vi "rs3 release frame.vi"(8 "error in (no error)":errorcluster, 11 "Frame":u64) -> (0 "error out":errorcluster, 3 "error":u64)   [LabVIEW 2018, in "libRealSense3.lvlib"]
doc: "You MUST release the FRAME handle soon after you are done with it. It does not have to be immediately, but within about 15 frames."
uses:
  libRealSense3.lvlib
  realsense2.dll
panel:
  # "RS3 Release Frame"
  # "(C) Intel Corp. 2017,  AGJ"
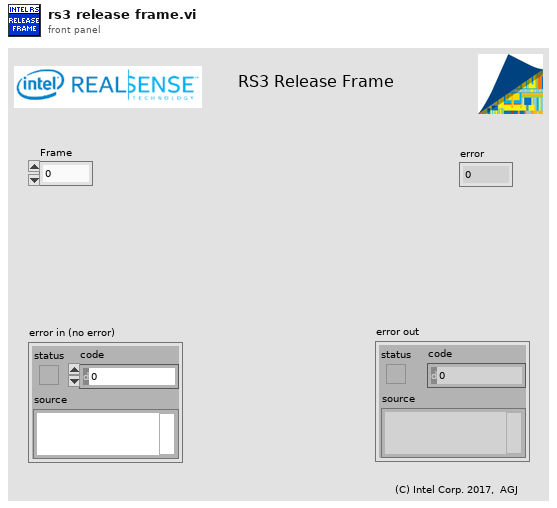
[diagram p1: front panel]
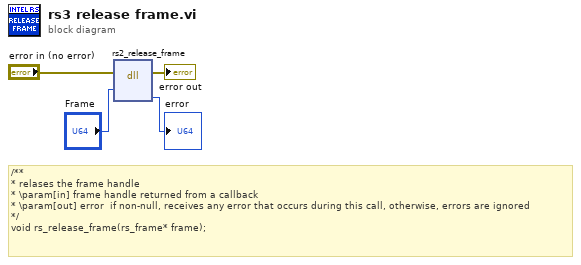
[diagram p0: block diagram]
diagram:
  # "/**\n* relases the frame handle\n* \\param[in] frame handle returned from a callback\n* \\param[out] error  if non-null, receives any error that occurs during this call, otherwise, errors are ignored\n*/\nvoid rs_release_frame(rs_frame* frame);"
  n1 = dll-call lib="C:/Users/aaron.jencks/Documents/Temp/realsense_labview_sdk/RealSense SDK2.11.0 for LabVIEW/realsense2.dll" fn="rs2_release_frame"(error in="error in (no error)", "frame"="Frame") -> (error out=→"error out":errorcluster, "error"=→"error":u64)  [unwired: 5 in, 1 out]
